vi "gfitsio-write-column-variant.vi"(4 "units":string, 6 "row":i32, 7 "column":string, 8 "error in (no error)":errorcluster, 9 "data":variant, 10 "Variable Size? (F)":bool, 11 "gfits refnum":T1) -> (0 "error out":errorcluster, 3 "dup gfits refnum":T1)   [LabVIEW 2022 SP3, in "gfitsio.lvlib"]
doc: "Write data to the table column (doing data type conversion if necessary). If the column does not exist, it is created using the parameters specified to this VI. If the row in which this data will be added does not exist it is appended to the table. If the row does exist then the cell is overwritten.\n\nThe FITS Standard recommends that only letters, digits, and the underscore character be used in column names (the ttype parameter) with no embedded spaces. Trailing blank characters are not significant. It is recommended that all the column names in a given table be unique within the first 8 characters, and strongly recommended that the names be unique within the first 16 characters.\n\nPhysical units are asscociated with the data in this column. GFITSIO writes this string to the FITS file the first time data is written to the column. If different units are supplied on a subsequent write GFITSIO will not overwrite the existing units."
uses:
  gfitsio.lvlib
  gfitsio-refnum.ctl
  gfitsio.dll
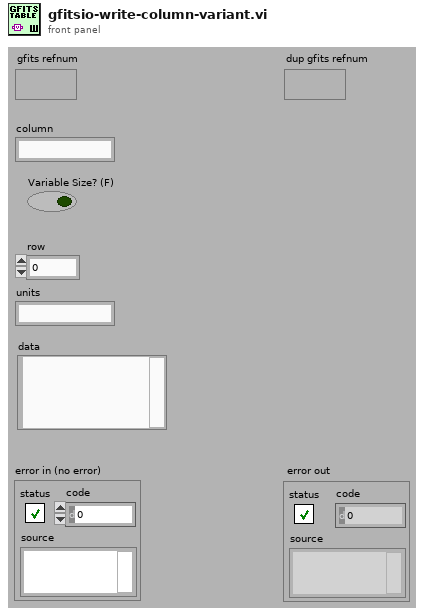
[diagram p1: front panel]
types:
  T1 = typedef "gfitsio.lvlib/gfitsio-refnum.ctl" = refnum<k1>
  T2 = typedef "gfitsio.lvlib/cfitsio-datatypes.ctl" = i32
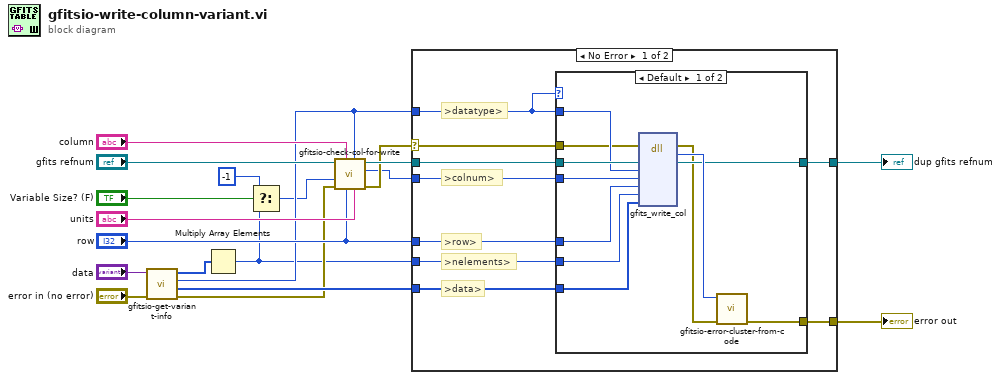
[diagram p0: block diagram]
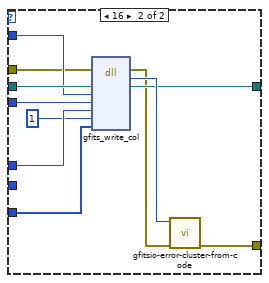
[diagram p2: hidden frame]
diagram:
  n1 = call "gfitsio-get-variant-info.vi"("error in (no error)"="error in (no error)", "variant"="data") -> ("error out"=w6:errorcluster, "data out"=w9:u8[], "cfitsio datatype"=w8:T2, "sizes"=w10:i32[])  [unwired: 6 in]
  n2 = Multiply Array Elements(1:w10) -> (0:w4:i32)
  n3 = Select(t=-1, s="Variable Size? (F)", f=w4) -> (s? t:f=w3:i32)
  n4 = call "gfitsio-check-col-for-write.vi"("units"="units", "cfitsio datatype"=w8, "row"="row", "column"="column", "error in (no error)"=w6, "size (-1:variable)"=w3, "gfits refnum"="gfits refnum") -> ("error out"=w15:errorcluster, "colnum"=w12:i32, "dup gfits refnum"=w16:T1)  [unwired: 2 out]
  n5 = case shown="No Error" w15 {
    selector: w15 -> [w21 w52]
    tunnel: [w28 w52] -> w18
    tunnel: w16 -> [w26 w51]
    tunnel: [w27 w51] -> w19
    tunnel: w12 -> [w25 _]
    tunnel: w8 -> [w20 _]
    tunnel: "row" -> [w24 _]
    tunnel: w9 -> [w23 _]
    tunnel: w4 -> [w22 _]
    frame No Error {
      # ">datatype>"
      # ">data>"
      # ">nelements>"
      # ">row>"
      # ">colnum>"
      n6 = case shown="Default" w20 {
        tunnel: [w39 w50] -> w28
        tunnel: [w37 w48] -> w27
        tunnel: w26 -> [w36 w47]
        tunnel: w25 -> [w35 w46]
        tunnel: w20 -> [w34 w45]
        tunnel: w24 -> [w33 w44]
        tunnel: w23 -> [w32 w43]
        tunnel: w22 -> [w31 _]
        tunnel: w21 -> [w30 w42]
        frame Default {
          n7 = dll-call lib="C:/Development/rimas/RIMAS/gfitsio/gfitsio.dll" fn="gfits_write_col"(error in=w30, "refnum"=w36, "datatype"=w34, "column"=w35, "row"=w33, "nelements"=w31, "data"=w32) -> (error out=w29:errorcluster, "return type"=w38:i32, "refnum"=w37:T1)  [unwired: 7 in, 1 out]
          n8 = call "gfitsio-error-cluster-from-code.vi"("error in (no error)"=w29, "error code"=w38) -> ("error out"=w39:errorcluster)  [unwired: 9 out]
        }
        frame 16 {
          n9 = dll-call lib="C:/Development/rimas/RIMAS/gfitsio/gfitsio.dll" fn="gfits_write_col"(error in=w42, "refnum"=w47, "datatype"=w45, "column"=w46, "row"=w44, "nelements"=1, "data"=w43) -> (error out=w41:errorcluster, "return type"=w49:i32, "refnum"=w48:T1)  [unwired: 7 in, 1 out]
          n10 = call "gfitsio-error-cluster-from-code.vi"("error in (no error)"=w41, "error code"=w49) -> ("error out"=w50:errorcluster)  [unwired: 9 out]
        }
      }
    }
    frame Error {
    }
  }
  "error out" <- w18
  "dup gfits refnum" <- w19
